vi "Test_server_port.vi"(0 "IP & Port No":string, 2 "timeout ms (60000)":i32=1000, 3 "error in (no error)":errorcluster) -> (6 "error out":errorcluster)   [LabVIEW 2010]
panel:
  out "connection ID":refnum<k5>
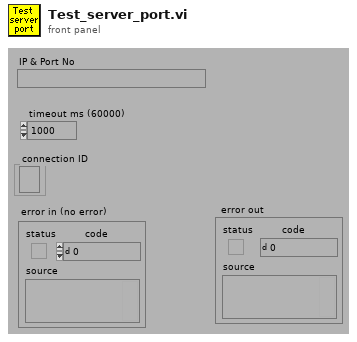
[diagram p1: front panel]
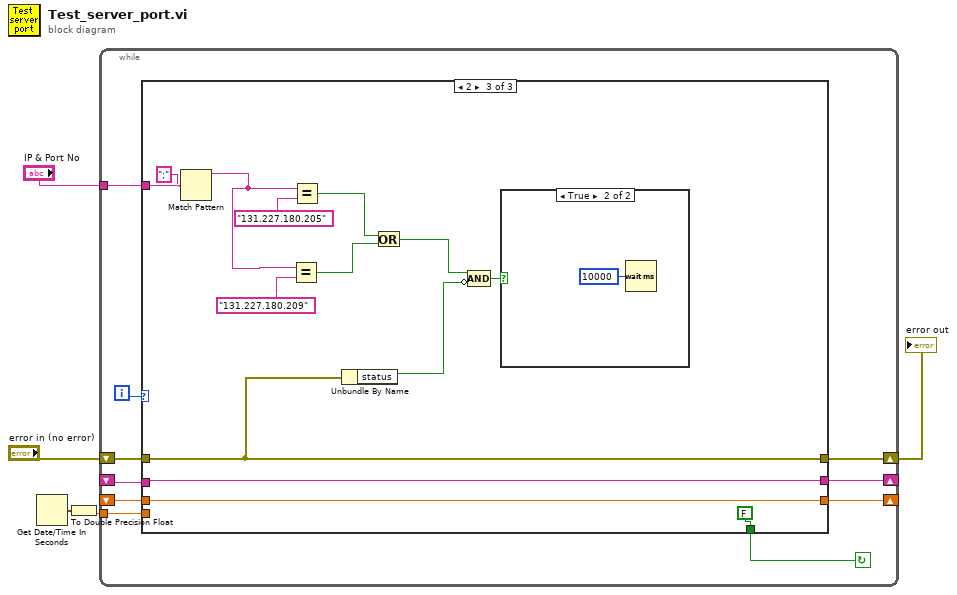
[diagram p0: block diagram]
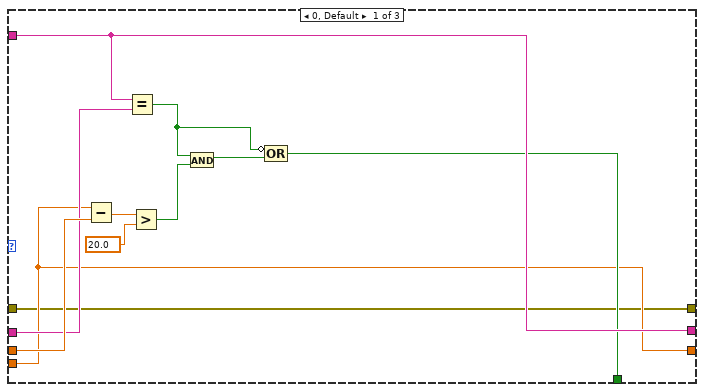
[diagram p2: hidden frame]
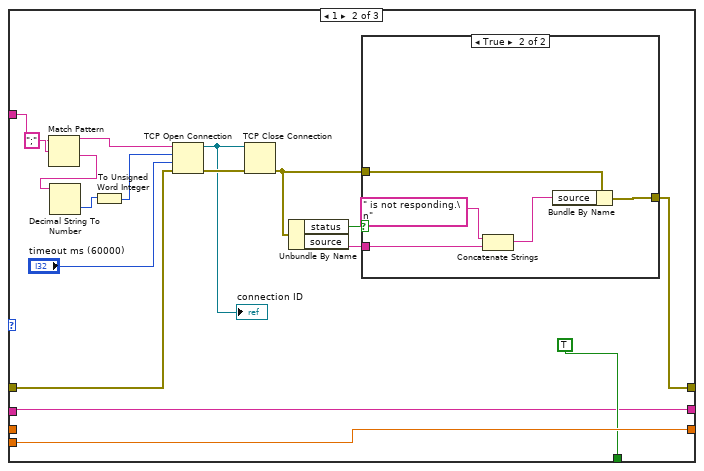
[diagram p3: hidden frame]
diagram:
  n1 = Get Date/Time In Seconds() -> (seconds since 1Jan1904=w1:timestamp)
  n2 = To Double Precision Float(number=w1) -> (double precision float=w4:dbl)
  n3 = while {
    shift-left: "error in (no error)" -> [w6]
    shift-right: [w7] -> w3
    tunnel: w4 -> [w12]
    shift-left: _ -> [w10]
    shift-right: [w13] -> _
    tunnel: "IP & Port No" -> [w14]
    shift-left: _ -> [w9]
    shift-right: [w11] -> _
    i -> [w15]
    stop <- w8 continue-if-true
    n4 = case shown="2" w15 {
      tunnel: [w16 w38 w59] -> w7
      tunnel: w14 -> [w23 w32 w56]
      tunnel: [w17 w37 w62] -> w13
      tunnel: w12 -> [w17 w37 _]
      tunnel: [w23 w35 w63] -> w11
      tunnel: w10 -> [w26 _ w62]
      tunnel: w9 -> [w22 w35 w63]
      tunnel: [w18 TRUE FALSE] -> w8
      tunnel: w6 -> [w16 w34 w59]
      frame 0, Default {
        n5 = Subtract(x=w17, y=w26) -> (x-y=w25:dbl)
        n6 = Equal?(x=w23, y=w22) -> (x = y?=w19:bool)
        n7 = Greater?(x=w25, y=20.0) -> (0:w21:bool)
        n8 = And(x=w19, y=w21) -> (x .and. y?=w20:bool)
        n9 = Compound Arithmetic op=OR(invert w19, w20) -> (w18:bool)
      }
      frame 1 {
        n10 = Match Pattern(string=w32, regular expression=";") -> (before substring=w28:string, after substring=w29:string)  [unwired: 3 out]
        n11 = Decimal String To Number(string=w29) -> (number=w31:i32)  [unwired: 3 out]
        n12 = To Unsigned Word Integer(number=w31) -> (unsigned 16bit integer=w30:u16)
        n13 = TCP Open Connection(address=w28, remote port or service name=w30, timeout ms (60000)="timeout ms (60000)", error in (no error)=w34) -> (connection ID=w41:refnum<k5>, error out=w42:errorcluster)  [unwired: 1 out]
        "connection ID" <- w41
        n14 = TCP Close Connection(connection ID=w41, error in (no error)=w42) -> (error out=w40:errorcluster)  [unwired: 2 out]
        n15 = Unbundle By Name(w40) -> ("status"=w39:bool, "source"=w27:string)
        n16 = case shown="True" w39 {
          tunnel: w40 -> [w44 w49]
          tunnel: [w44 w48] -> w38
          tunnel: w27 -> [_ w46]
          frame False {
          }
          frame True {
            n17 = Concatenate Strings(" is not responding.\n" ("Format String"), w46) -> (w45:string)
            n18 = Bundle By Name(cluster=w49, "source"=w45) -> (w48:errorcluster)
          }
        }
      }
      frame 2 {
        n19 = Match Pattern(string=w56, regular expression=";") -> (before substring=w53:string)  [unwired: 4 out]
        n20 = Equal?(x=w53, y="131.227.180.209") -> (x = y?=w52:bool)
        n21 = Equal?(x=w53, y="131.227.180.205") -> (x = y?=w51:bool)
        n22 = Unbundle By Name(w59) -> ("status"=w58:bool)
        n23 = Or(x=w51, y=w52) -> (x .or. y?=w50:bool)
        n24 = Compound Arithmetic op=AND(w50, invert w58) -> (w57:bool)
        n25 = case shown="True" w57 {
          frame False {
          }
          frame True {
            n26 = Wait (ms)(milliseconds to wait=u32 10000) -> ()  [unwired: 1 out]
          }
        }
      }
    }
  }
  "error out" <- w3
